vi "Enable Limit Test Auto Clear.vi"(0 "VISA resource name":refnum<visa-resource-name>, 5 "Function":u16(ring) items=["Voltage: DC", "Voltage: AC", "Current: DC", "Current: AC", "2W Resistance", "4W Resistance", "Diode", "Capacitance", "Temperature", "Continuity", "Frequency", "Period", "Ratio", "Digitize Voltage", "Digitize Current"], 7 "Limit Test Number":u16 min=1 max=2 step=1, 9 "Enable Limit Test Auto Clear":bool, 11 "error in (no error)":errorcluster) -> (4 "VISA resource name out":refnum<visa-resource-name>, 15 "error out":errorcluster)   [LabVIEW 2009, in "Keithley DMM7510.lvlib"]
doc: "This VI configures if limit Y should be cleared automatically or not."
uses:
  Keithley DMM7510.lvlib
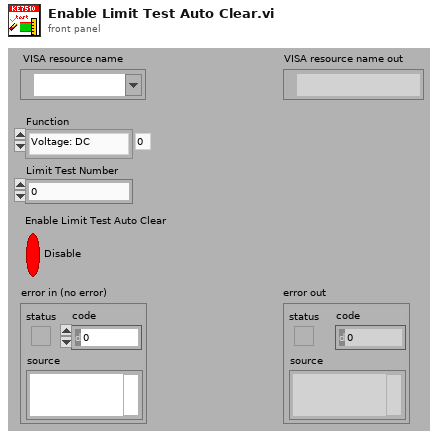
[diagram p1: front panel]
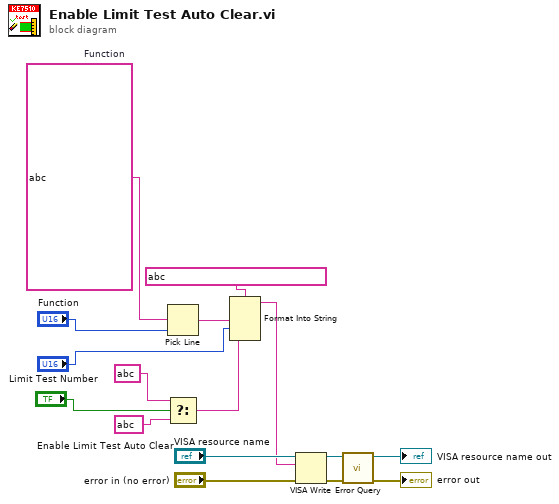
[diagram p0: block diagram]
diagram:
  w7 = string ?  # Function
  n1 = Pick Line(multi-line string=w7, line index="Function") -> (output string=w8:string)  [unwired: 1 out]
  n2 = Select(t=string ? ("format string"), s="Enable Limit Test Auto Clear", f=string ? ("format string")) -> (s? t:f=w1:string)
  n3 = Format Into String(format string=string ?, w8, "Limit Test Number", w1) -> (resulting string=w9:string)  [unwired: 2 in, 1 out]
  n4 = VISA Write(VISA resource name="VISA resource name", write buffer=w9, error in (no error)="error in (no error)") -> (VISA resource name out=w12:refnum<visa-resource-name>, error out=w11:errorcluster)  [unwired: 1 out]
  n5 = call "Error Query.vi"("error in (no error)"=w11, "VISA resource name"=w12) -> ("error out"=→"error out":errorcluster, "VISA resource name out"=→"VISA resource name out":refnum<visa-resource-name>)  [unwired: 8 out]
